vi "Analog Output - N Channels - 1 Sample.vi"() -> ()   [LabVIEW 2019]
uses:
  <vilib>/myRIO/Common/Instrument Driver Framework/ELVIS III v1.0/AO/vis/ELVIS III v1.0 Close AO.vi
  <vilib>/myRIO/Common/Instrument Driver Framework/myRIO v1.0/UART/vis/myRIO v1.0 Close UART.vi
  <vilib>/myRIO/Common/Instrument Driver Framework/ELVIS III v1.0/AO/vis/ELVIS III v1.0 Unreserve AO.vi
  <vilib>/myRIO/Common/Instrument Driver Framework/ELVIS III v1.0/AO/vis/ELVIS III v1.0 Build MUX Configuration AO.vi
  <vilib>/Utility/error.llb/Error Cluster From Error Code.vi
  <vilib>/myRIO/Common/Instrument Driver Framework/ELVIS III v1.0/AO/vis/ELVIS III v1.0 Write AO.vi
  <vilib>/myRIO/Common/Instrument Driver Framework/ELVIS III v1.0/Resource Manager/vis/ELVIS III v1.0 Unreserve Channel List.vi
  <vilib>/myRIO/Common/Instrument Driver Framework/myRIO v1.0/myRIO v1.0 Close.vi
  <vilib>/myRIO/Common/Instrument Driver Framework/Utilities/vis/FPGA Ref Manager.vi
  <vilib>/myRIO/Common/Instrument Driver Framework/ELVIS III v1.0/ELVIS III v1.0 Reset FPGA.vi
  <vilib>/myRIO/Common/Instrument Driver Framework/myRIO v1.0/IRQ/vis/myRIO v1.0 IRQ Info FGV.vi
  <vilib>/myRIO/Common/Instrument Driver Framework/myRIO v1.0/IRQ/vis/myRIO v1.0 Timer IRQ Info FGV.vi
  <vilib>/myRIO/Common/Instrument Driver Framework/myRIO v1.0/IRQ/vis/myRIO v1.0 ISR Agent.vi
  <vilib>/myRIO/Instrument Drivers/Utilities/vis/Reset Index.vi
  <vilib>/myRIO/Common/Instrument Driver Framework/myRIO v1.0/Resource Manager/vis/myRIO v1.0 Block Write Resource Manager.vi
  <vilib>/myRIO/Instrument Drivers/Utilities/Utilities.lvlib
  <vilib>/myRIO/Instrument Drivers/Onboard IO/AO/AO.lvlib
panel:
  in  "Stop":bool
  in  "A/AO1 (V)":dbl min=-10.0 max=10.0 step=0.1 format="%#_13g"
  in  "A/AO0 (V)":dbl min=-10.0 max=10.0 step=0.1 format="%#_13g"
  # "ELVIS III Control IO"
  # "模拟输出N通道"
  # "Overview: Outputs specified voltage values on Bank A, Channels AO0 and AO1 (A/AO0 and A/AO1).\nInstructions:\n1. Select initial output voltage values below.\n2. Connect A/AO0 to the positive lead of one load, and connect AGND to the negative lead of the same load. Connect A/AO1 to the positive lead of another load, and connect AGND to the negative lead of the corresponding load. AGND is the ground reference terminal for analog output channels.\n3. Run the VI.\n4. Modify the analog output values.\n5. Press the Stop button to stop the VI."
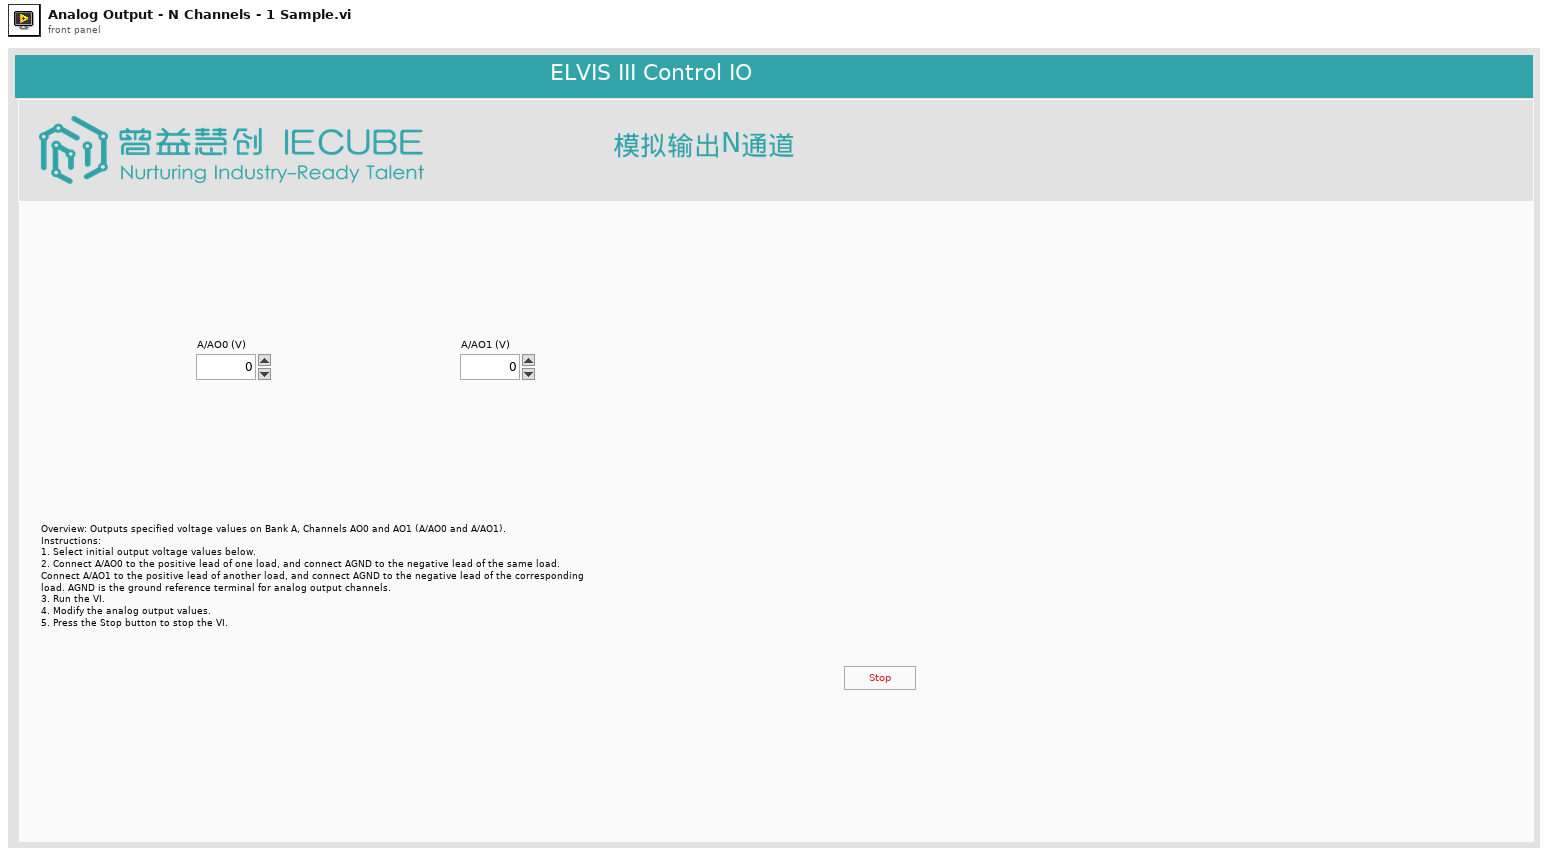
[diagram p1: front panel]
types:
  T1 = typedef "AO.lvlib/AO Reference.ctl" = cluster{"myRIO Reference":T2, "AO Channel List":T6, "AO Scaling Constant List":T8}
  T2 = typedef "myRIO Generic Hardware Reference.ctl" = cluster{"myRIO Model":T3, "myRIO Hardware Reference":T4}
  T3 = typedef "Hardware Version Enum.ctl" = enum16{"Unknown", "myRIO-1900", "myRIO-1950", "roboRIO", "NI ELVIS RIO CM", "ELVIS III"}
  T4 = typedef "myRIO v1.0 Reference.ctl" = cluster{"Generic FPGA Reference":T5, "Allow multiple opens":bool}
  T5 = typedef "Generic FPGA Reference.ctl" = refnum<k20>
  T6 = typedef "AO Channels List.ctl" = T7[]
  T7 = typedef "AO Channels Enum.ctl" = enum16{"Not Connected", "AudioOut/Left", "AudioOut/Right", "C/AO0", "C/AO1", "A/AO0", "A/AO1", "B/AO0", "B/AO1"}
  T8 = typedef "Analog Scaling Constants List.ctl" = T9[]
  T9 = typedef "Analog Scaling Constants.ctl" = cluster{"LSB Weight (Volts)":dbl, "Offset (Volts)":dbl, "Signed?":bool}
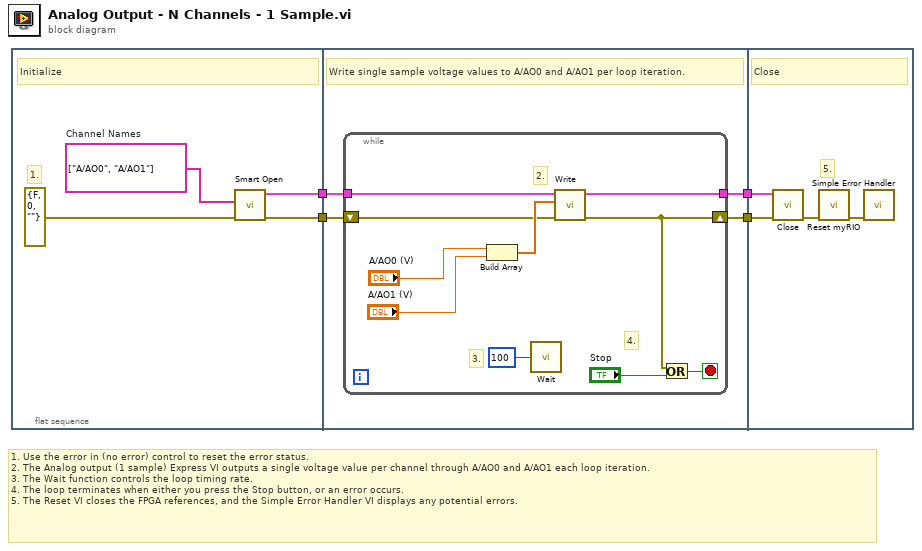
[diagram p0: block diagram]
diagram:
  # "1. Use the error in (no error) control to reset the error status. \n2. The Analog output (1 sample) Express VI outputs a single voltage value per channel through A/AO0 and A/AO1 each loop iteration.\n3. The Wait function controls the loop timing rate.\n4. The loop terminates when either you press the Stop button, or an error occurs.\n5. The Reset VI closes the FPGA references, and the Simple Error Handler VI displays any potential errors."
  n1 = flat-sequence {
    tunnel: [w7] -> w3
    tunnel: [w5] -> w2
    tunnel: [w12] -> w4
    tunnel: w3 -> [w11]
    tunnel: w2 -> [w10]
    tunnel: [w9] -> w1
    tunnel: w4 -> [w25]
    tunnel: w1 -> [w23]
    frame #0 {
      w8 = tag[] ["A/AO0", "A/AO1"]  # Channel Names
      # "1."
      # "Initialize"
      n2 = call <vilib>:"Smart Open.vi"("error in (no error)"=errorcluster {"status"=FALSE, "code"=0, "source"=""} ("Error In"), "Channel Names"=w8) -> ("error out"=w7:errorcluster, "AO Ref Out"=w5:T1)  [unwired: 8 in]
    }
    frame #1 {
      # "Write single sample voltage values to A/AO0 and A/AO1 per loop iteration."
      n3 = while {
        shift-right: [w17] -> w12
        shift-left: w11 -> [w18]
        tunnel: w10 -> [w14]
        tunnel: [w13] -> w9
        stop <- w22 stop-if-true
        # "4."
        # "3."
        # "2."
        n4 = Build Array("A/AO0 (V)", "A/AO1 (V)") -> (w19:dbl[])
        n5 = call "Wait"("Count(mSec)"=u32 100) -> ()  [unwired: 1 out]
        n6 = call <vilib>:"Write.vi"("error in (no error)"=w18, "Values"=w19, "AO Ref In"=w14) -> ("error out"=w17:errorcluster, "AO Ref Out"=w13:T1)  [unwired: 6 in]
        n7 = Or(x=w17, y="Stop") -> (x .or. y?=w22:bool)
      }
    }
    frame #2 {
      # "5."
      # "Close"
      n8 = call <vilib>:"Close.vi"("error in (no error)"=w25, "AO Ref In"=w23) -> ("error out"=w24:errorcluster)  [unwired: 9 in]
      n9 = call <vilib>:"Reset myRIO.vi"("error in (no error)"=w24) -> ("error out"=w26:errorcluster)  [unwired: 10 in]
      n10 = call <vilib>:"Simple Error Handler.vi"("error in (no error)"=w26) -> ()  [unwired: 4 in, 5 out]
    }
  }
